vi "UpdateArmState.vi"(8 "error in (no error)":errorcluster) -> ()   [LabVIEW 2015]
uses:
  Implementation/Shooter Global.vi
panel:
  out "Count":dbl
  out "Encoder Pos":dbl(graph)
  out "Current":dbl(graph)
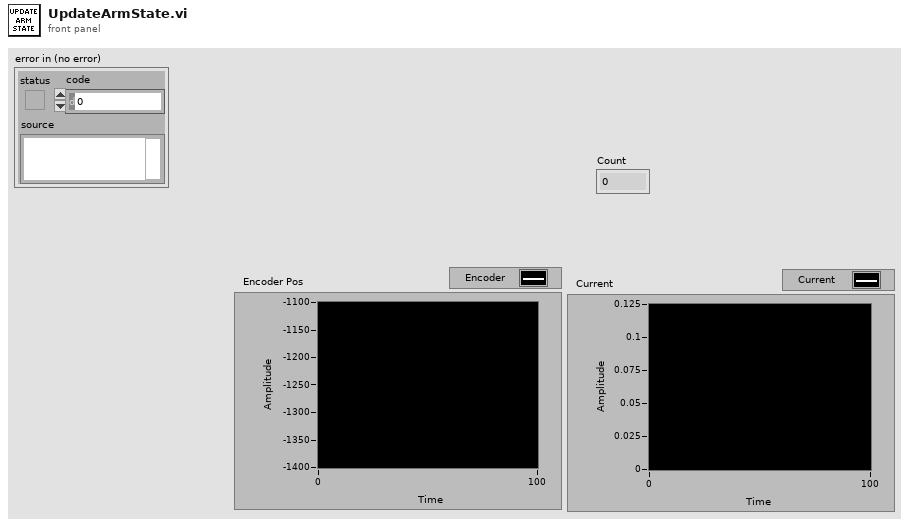
[diagram p1: front panel]
types:
  T1 = typedef "Detailed Motor Type Def.ctl" = cluster{"MotorRef":T2, "Encoder Ticks Per Rev":dbl, "Set Position":dbl, "Wheel Radius":dbl}
  T2 = typedef "WPI_MotorControlDeviceRef.ctl" = cluster{"DeviceStatus":errorcluster, "Type":T3, "PWM":cluster{"PWM Channel":T4, "DeadBand":T5}, "CAN":cluster{"Device Number":u8, "Control Mode":T6, "Semaphore":T7, "Max Vout":dbl, "TalonSRX Control Mode":T8}, "Invert":bool}
  T3 = typedef "WPI_MotorControlType.ctl" = enum16{"PWM", "CAN", "CANTalonSRX"}
  T4 = typedef "FPGA_DIOPWMChannel.ctl" = enum8{"PWM 0", "PWM 1", "PWM 2", "PWM 3", "PWM 4", "PWM 5", "PWM 6", "PWM 7", "PWM 8", "PWM 9", "PWM MXP 0", "PWM MXP 1", "PWM MXP 2", "PWM MXP 3", "PWM MXP 4", "PWM MXP 5", "PWM MXP 6", "PWM MXP 7", "PWM MXP 8", "PWM MXP 9", "Invalid"}
  T5 = typedef "WPI_PWMDeadband.ctl" = cluster{"Name":string, "maxPositivePwm":i32, "minPositivePwm":i32, "centerPwm":i32, "maxNegativePwm":i32, "minNegativePwm":i32, "angularRange":u16}
  T6 = typedef "WPI_CANJaguar_ControlMode.ctl" = enum8{"Percent VBus", "Current", "Speed", "Position", "Voltage"}
  T7 = typedef "Semaphore RefNum" = refnum<k1>
  T8 = typedef "WPI_CANTalonSRX_APIControlMode.ctl" = enum8{"Percent VBus", "Speed", "Position", "Slave", "Unchanged / Invalid", "Voltage Compensation", "Current", "Motion Profile"}
  T9 = typedef "Arm Settings Type Def.ctl" = cluster{"Min Arm Pos":dbl, "Max Arm Pos":dbl, "Drive Pos":dbl, "Arm Increments":dbl, "Obstacle Pos":dbl, "Max Current":dbl}
  T10 = typedef "WPI_CANTalonSRX_GlobalStatus.ctl" = cluster{"Applied Throttle":dbl, "Module Enabled":bool, "CAN Error":errorcluster, "Closed Loop Error":dbl, "Forward Limit Switch Closed":bool, "Reverse Limit Switch Closed":bool, "Sensor Position":dbl, "Sensor Velocity":dbl, "Current":dbl, "Sticky Fault - Over Temp":bool, "Sticky Fault - Under Voltage":bool, "Sticky Fault - Forward Limit":bool, "Sticky Fault - Reverse Limit":bool, "Sticky Fault - Forward Soft Limit":bool, "Sticky Fault - Reverse Soft Limit":bool, "Brake is Enabled":bool, "Encoder Position":dbl, "Encoder Velocity":dbl, "Encoder Index Count":dbl, "Encoder A Pin State":bool, "Encoder B Pin State":bool, "Encoder Index Pin State":bool, "Analog In":dbl, "Analog In Velocity":dbl, "Temperature (C)":dbl, "Battery Voltage":dbl, "Control 5 Is Supported":bool, "Current Profile Slot Select":dbl, "Pos Div 8":bool, "Vel Div 4":bool, "Pulse Width Position":i32, "Pulse Width Velocity":i32, "Pulse Width Rise To Rise (us)":i32, "Pulse Width Rise To Fall (us)":i32, "Mot Prof Active Is Under Run":bool, "Mot Prof Active Has Under Run":bool, "Mot Prof Active Is Last":bool, "Mot Prof Active Velocity Only":bool, "Mot Prof Active Is Valid":bool, "Mot Prof Buffer Is Full":bool, "Mot Prof Active Profile Slot Select":i32, "Mot Prof NextID":i32, "Mot Prof Count":i32, "Mot Prof Active Velocity":dbl, "Mot Prof Active Position":dbl, "Mot Prof Output Enable":i32}
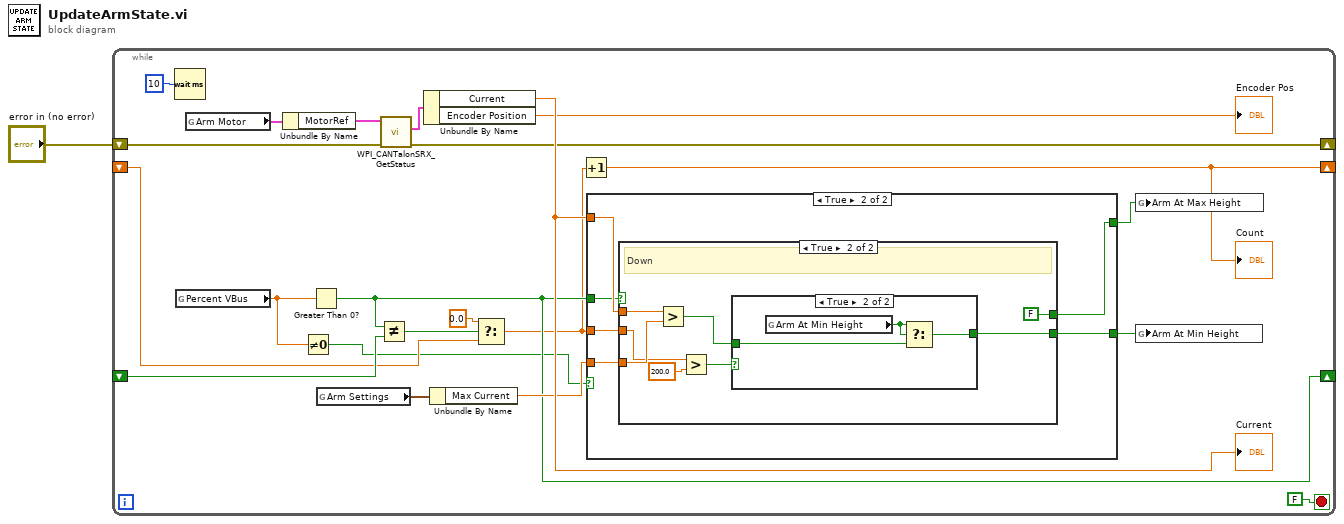
[diagram p0: block diagram]
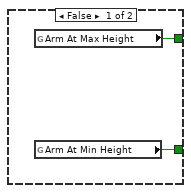
[diagram p2: hidden frame]
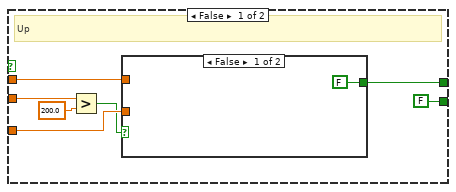
[diagram p3: hidden frame]
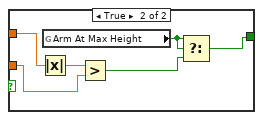
[diagram p4: hidden frame]
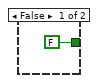
[diagram p5: hidden frame]
diagram:
  n1 = while {
    shift-right: [w11] -> _
    shift-left: "error in (no error)" -> [w12]
    shift-right: [w5] -> _
    shift-left: _ -> [w6]
    shift-right: [w10] -> _
    shift-left: _ -> [w9]
    stop <- FALSE stop-if-true
    n2 = Wait (ms)(milliseconds to wait=u32 10) -> ()  [unwired: 1 out]
    n3 = global read "Shooter Global.vi" "Percent VBus"() -> (w2:dbl)
    n4 = global read "Shooter Global.vi" "Arm Motor"() -> (w22:T1)
    n5 = Unbundle By Name(w22) -> ("MotorRef"=w21:T2)
    n6 = Not Equal To 0?(x=w2) -> (x != 0?=w3:bool)
    n7 = Greater Than 0?(x=w2) -> (x > 0?=w10:bool)
    n8 = global read "Shooter Global.vi" "Arm Settings"() -> (w17:T9)
    n9 = Not Equal?(x=w10, y=w9) -> (x != y?=w8:bool)
    n10 = call <vilib>:"WPI_CANTalonSRX_GetStatus.vi"("error in (no error)"=w12, "CAN Talon SRX Ref"=w21) -> ("error out"=w11:errorcluster, "Talon SRX Status"=w23:T10)  [unwired: 7 in, 1 out]
    n11 = Unbundle By Name(w23) -> ("Current"=w18:dbl, "Encoder Position"=→"Encoder Pos":dbl)
    "Current" <- w18
    n12 = Unbundle By Name(w17) -> ("Max Current"=w16:dbl)
    n13 = Select(t=0.0, s=w8, f=w6) -> (s? t:f=w4:dbl)
    n14 = Increment(x=w4) -> (x+1=w5:dbl)
    "Count" <- w5
    n15 = case shown="True" w3 {
      tunnel: w18 -> [_ w31]
      tunnel: w16 -> [_ w30]
      tunnel: [w24 w29] -> w14
      tunnel: [w25 w28] -> w13
      tunnel: w10 -> [_ w27]
      tunnel: w4 -> [_ w26]
      frame False {
        n16 = global read "Shooter Global.vi" "Arm At Max Height"() -> (w24:bool)
        n17 = global read "Shooter Global.vi" "Arm At Min Height"() -> (w25:bool)
      }
      frame True {
        n18 = case shown="True" w27 {
          tunnel: w31 -> [w35 w49]
          tunnel: w30 -> [w36 w50]
          tunnel: [w37 FALSE] -> w29
          tunnel: [FALSE w51] -> w28
          tunnel: w26 -> [w32 w47]
          frame False {
            # "Up"
            n19 = Greater?(x=w32, y=200.0) -> (0:w33:bool)
            n20 = case shown="False" w33 {
              tunnel: [FALSE w44] -> w37
              tunnel: w36 -> [_ w43]
              tunnel: w35 -> [_ w41]
              frame False {
              }
              frame True {
                n21 = Absolute Value(x=w41) -> (abs(x)=w40:dbl)
                n22 = global read "Shooter Global.vi" "Arm At Max Height"() -> (w45:bool)
                n23 = Greater?(x=w40, y=w43) -> (0:w42:bool)
                n24 = Select(t=w45, s=w45, f=w42) -> (s? t:f=w44:bool)
              }
            }
          }
          frame True {
            # "Down"
            n25 = Greater?(x=w49, y=w50) -> (0:w52:bool)
            n26 = Greater?(x=w47, y=200.0) -> (0:w48:bool)
            n27 = case shown="True" w48 {
              tunnel: w52 -> [_ w56]
              tunnel: [FALSE w55] -> w51
              frame False {
              }
              frame True {
                n28 = global read "Shooter Global.vi" "Arm At Min Height"() -> (w57:bool)
                n29 = Select(t=w57, s=w57, f=w56) -> (s? t:f=w55:bool)
              }
            }
          }
        }
      }
    }
    n30 = global write "Shooter Global.vi" "Arm At Max Height"(w14) -> ()
    n31 = global write "Shooter Global.vi" "Arm At Min Height"(w13) -> ()
  }
